vi "LogToSyslog.vi"(5 "call chain level (1)":i32=1, 7 "severity (informational)":i32(ring)=2 items=["Error", "Warning", "Informational"], 10 "error in (no error)":errorcluster, 11 "message":string) -> (2 "error out":errorcluster, 3 "Syslog Message":string)   [LabVIEW 2020, in "VsDebugLibrary.lvlib"]
uses:
  VsDebugLibrary.lvlib
  <vilib>/Utility/SystemLogging/NI_SystemLogging.lvlib
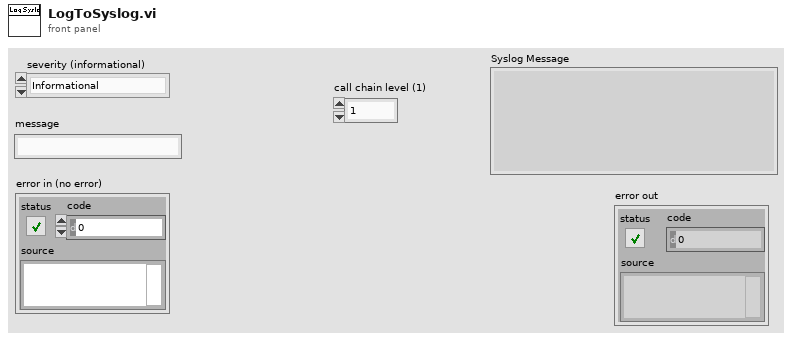
[diagram p1: front panel]
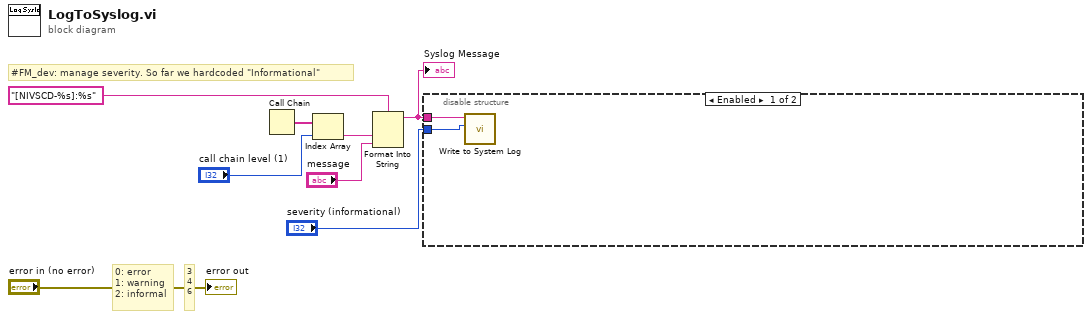
[diagram p0: block diagram]
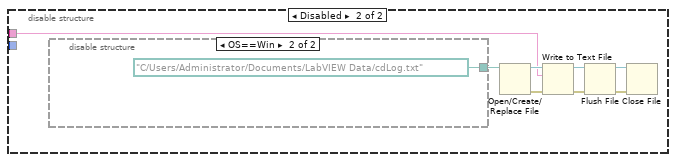
[diagram p2: hidden frame]
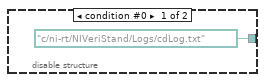
[diagram p3: hidden frame]
diagram:
  # "3\n4\n6"
  # "0: error\n1: warning\n2: informal"
  # "#FM_dev: manage severity. So far we hardcoded \"Informational\""
  n1 = Call Chain() -> (call chain=w4:string[])
  n2 = Index Array(array=w4, index="call chain level (1)") -> (element=w1:string)
  n3 = Format Into String(format string="[NIVSCD-%s]:%s", w1, "message") -> (resulting string=w5:string)  [unwired: 2 in, 1 out]
  "Syslog Message" <- w5
  n4 = disable-structure shown="Enabled" {
    disable-tunnel: "severity (informational)" -> [w10 _]
    disable-tunnel: w5 -> [w9 w11]
    frame Enabled {
      n5 = call <vilib>:"Write to System Log.vi"("severity"=w10, "message"=w9) -> ()  [unwired: 9 in, 1 out]
    }
    frame Disabled {
      n6 = disable-structure shown="OS==Win" {
        disable-tunnel: [path "c:/ni-rt/NIVeriStand/Logs/cdLog.txt" ("file path (use dialog)") path "C:/Users/Administrator/Documents/LabVIEW Data/cdLog.txt" ("file path (use dialog)")] -> w18
        frame condition #0 {
        }
        frame condition #1 (active) {
        }
      }
      n7 = Open/Create/Replace File(file path (use dialog)=w18) -> (refnum out=w17:refnum<file>, error out=w16:errorcluster)  [unwired: 5 in, 1 out]
      n8 = Write to Text File(file (use dialog)=w17, text=w11, error in=w16) -> (refnum out=w14:refnum<file>, error out=w15:errorcluster)  [unwired: 1 in, 1 out]
      n9 = Flush File(refnum=w14, error in=w15) -> (refnum out=w13:refnum<file>, error out=w12:errorcluster)
      n10 = Close File(refnum=w13, error in=w12) -> ()  [unwired: 2 out]
    }
  }
  "error out" <- "error in (no error)"
